vi "The_Cat_Escape.vi"() -> ()   [LabVIEW 2019]
panel:
  out "Boolean":bool
  in  "stop":bool
  in  "Left":i64(slide) scale=-200.0..200.0
  in  "Top":i64(slide) scale=200.0..-200.0
  in  "Cat":enum32{"Page 1", "Page 2"}(tab)
  # "MOVE USING THESE\n<-----"
  # "Your goal is to help the Cat escape the box by using the sliders.\n\nWhen the cat is entirely outside of the box, the Boolean LED should light up. When the program starts, the cat should reset back to the middle of the box and the LED should be off."
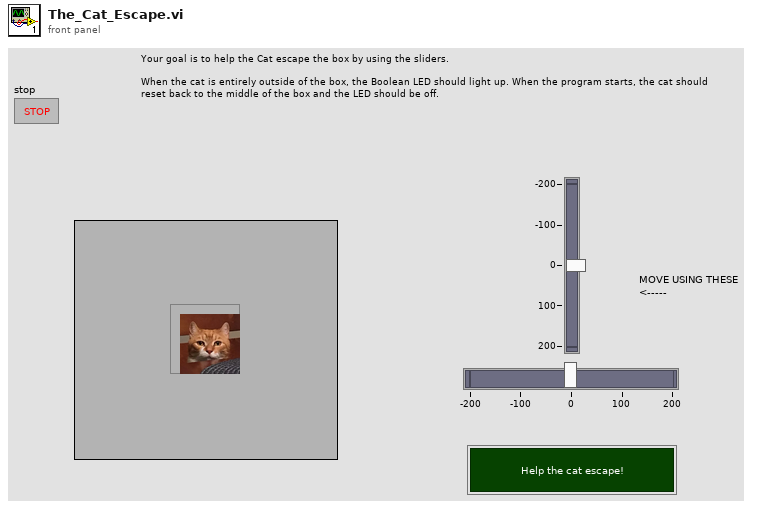
[diagram p1: front panel]
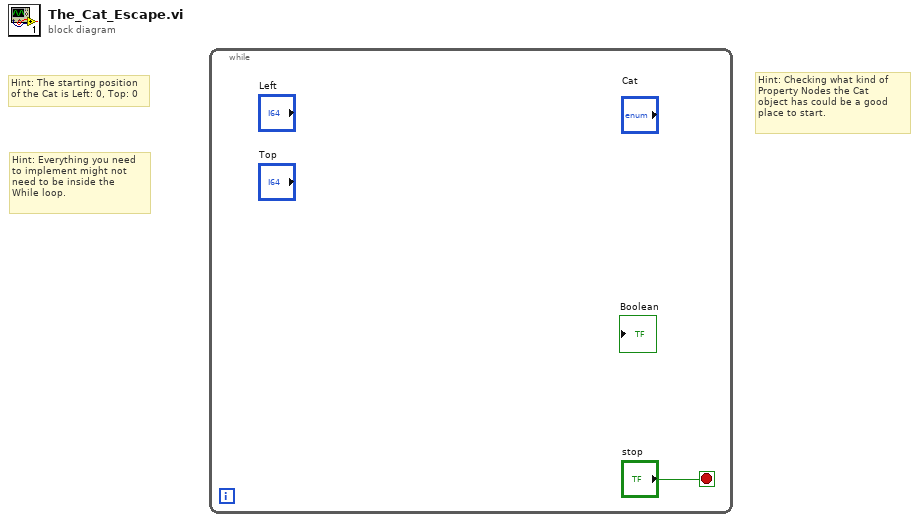
[diagram p0: block diagram]
diagram:
  # "Hint: The starting position\nof the Cat is Left: 0, Top: 0"
  # "Hint: Everything you need\nto implement might not \nneed to be inside the \nWhile loop."
  # "Hint: Checking what kind of \nProperty Nodes the Cat \nobject has could be a good\nplace to start."
  n1 = while {
    stop <- "stop" stop-if-true
  }
